vi "LabVIEW2020串口通信.vi"() -> ()   [LabVIEW 2020]
uses:
  <vilib>/Instr/_visa.llb/VISA Configure Serial Port (Instr).vi
panel:
  in  "STOP":bool
  out "读取缓冲区":string
  in  "OK":bool
  in  "写入缓冲区":string
  in  "VISA资源名称":refnum<visa-resource-name>
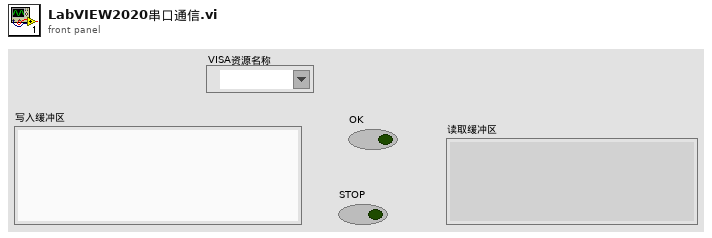
[diagram p1: front panel]
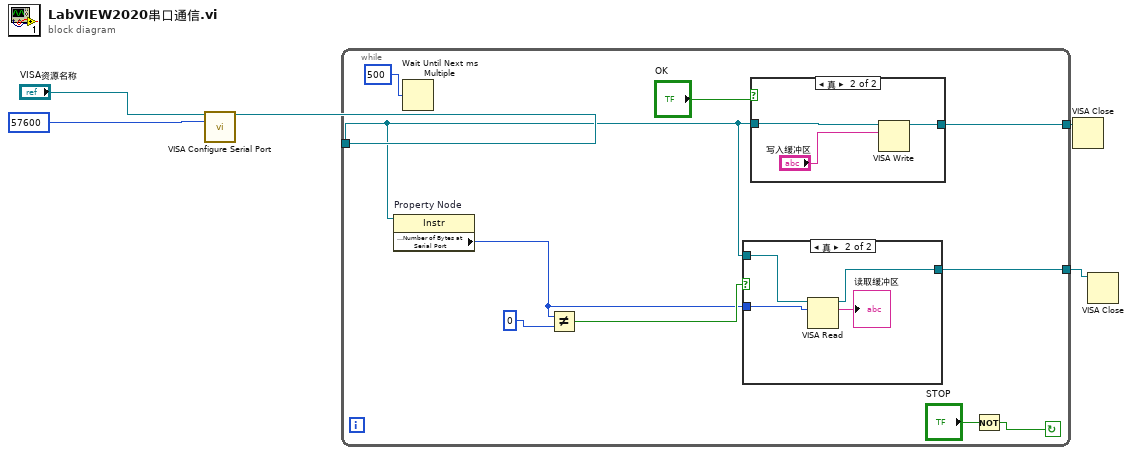
[diagram p0: block diagram]
diagram:
  n1 = call-poly "VISA Configure Serial Port"("VISA resource name"="VISA资源名称", "baud rate (9600)"=u32 57600) -> ("VISA resource name out"=w3:refnum<visa-resource-name>)  [unwired: 12 in, 1 out]
  n2 = while {
    tunnel: w3 -> [w13]
    tunnel: [w10] -> w2
    tunnel: [w9] -> w1
    stop <- w6 continue-if-true
    n3 = property on="Property Node" class="Instr"(reference=w13) -> ("Serial Settings:Number of Bytes at Serial Port"=w7:u32)  [unwired: 1 in, 2 out]
    n4 = Wait Until Next ms Multiple(millisecond multiple=u32 500 ("毫秒计时值")) -> ()  [unwired: 1 out]
    n5 = Not Equal?(x=w7, y=0) -> (x != y?=w11:bool)
    n6 = case shown="真" w11 {
      tunnel: w13 -> [w20 w24]
      tunnel: [w20 w22] -> w9
      tunnel: w7 -> [_ w21]
      frame False {
      }
      frame True {
        n7 = VISA Read(VISA resource name=w24, byte count=w21) -> (VISA resource name out=w22:refnum<visa-resource-name>, read buffer=→"读取缓冲区":string)  [unwired: 1 in, 2 out]
      }
    }
    n8 = case shown="真" "OK" {
      tunnel: w13 -> [w16 w19]
      tunnel: [w16 w17] -> w10
      frame False {
      }
      frame True {
        n9 = VISA Write(VISA resource name=w19, write buffer="写入缓冲区") -> (VISA resource name out=w17:refnum<visa-resource-name>)  [unwired: 1 in, 2 out]
      }
    }
    n10 = Not(x="STOP") -> (.not. x?=w6:bool)
  }
  n11 = VISA Close(VISA resource name=w2) -> ()  [unwired: 1 in, 1 out]
  n12 = VISA Close(VISA resource name=w1) -> ()  [unwired: 1 in, 1 out]
